vi "example 8 - grand child.vi"() -> ()   [LabVIEW 2020]
panel:
  in  "n-label-unvis":bool
  in  "n-label-vis":bool
  in  "m-label-vis":bool
  in  "m-label-unvis":bool
  in  "Reset":bool
  out "String":string
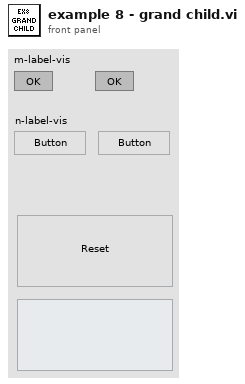
[diagram p1: front panel]
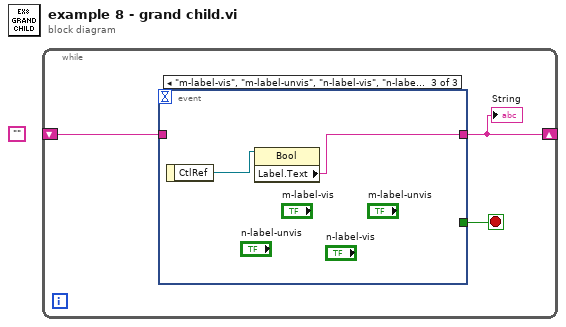
[diagram p0: block diagram]
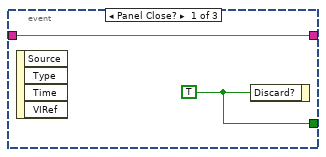
[diagram p2: hidden frame]
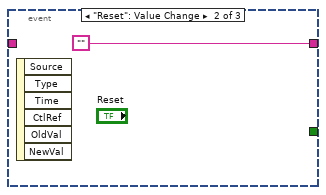
[diagram p3: hidden frame]
diagram:
  (unwired) ""
  n1 = while {
    shift-right: [w1] -> _
    shift-left: _ -> [w2]
    stop <- w3 stop-if-true
    n2 = event shown="[2] \"m-label-vis\", \"m-label-unvis\", \"n-label-vis\", \"n-label-unvis\": Value Change" {
      selector: _ -> [_ _ _]
      dyn-events: _ -> [_ _ _]
      timeout: _ -> [_ _ _]
      tunnel: [w5 _ _] -> w3
      tunnel: [w4 "" w7] -> w1
      tunnel: w2 -> [w4 _ _]
      event Panel Close? {
        w5 = TRUE
        n3 = event-data() -> ()  [unwired: 1 in, 4 out]
        n4 = event-data("Discard?"=w5) -> ()  [unwired: 1 in, 1 out]
      }
      event "Reset": Value Change {
        n5 = event-data() -> ()  [unwired: 1 in, 6 out]
      }
      event "m-label-vis", "m-label-unvis", "n-label-vis", "n-label-unvis": Value Change {
        n6 = event-data() -> ("CtlRef"=w8:refnum<vi>)  [unwired: 1 in]
        n7 = property class="Bool"(reference=w8) -> ("Label.Text"=w7:string)  [unwired: 1 in, 2 out]
      }
    }
    "String" <- w1
  }
